vi "Set Controls Enable or Disable State Crop Utility.vi"(8 "error in (no error)":errorcluster, 10 "State":T1, 11 "Frame Grabber Data In":T2={"Camera Session"="", "Frame"=refnum, "AVI Refnum"=refnum, "Codecs"=[], "Frame number"=0, "Tracking File Refnum"=refnum, "Tick Count"=0, "Probe Object"=refnum, "Playback Probe Data"=[], "Rigid Body"={"Position"={"x (mm)"=0.0, "y (mm)"=0.0, "z (mm)"=0.0}, "Orientation"={"Pitch (rad)"=0.0, "Yaw (rad)"=0.0, "Roll (rad)"=0.0}, "Quaternion"={"qx"=0.0, "qy"=0.0, "qz"=0.0, "qw"=0.0}, "Tracked?"=FALSE}, "Total no frames playback"=0, "Video FPS"=0.0, "Camera connected?"=FALSE, "Scene"=refnum, "Cropped Frame"=refnum, "Tracker FPS"=0.0, "Crop ROI"=[], "Presentation Values"=[], "Elapsed time (ms)"=0, "Camera frames playback"=0, "Refnums"={"Live Refnum"=refnum, "Record Refnum"=refnum, "Playback Refnum"=refnum, "Frame Slider Refnum"=refnum, "Pause Refnum"=refnum, "Home Refnum"=refnum, "Set Crop Refnum"=refnum, "Clear Crop Refnum"=refnum, "stop refnum"=refnum, "Playback Rate Refnum"=refnum, "Presentation Refnum"=refnum, "Crop Time Frame Slider Refnum"=refnum, "Cancel Save Refnum"=refnum, "Reverse Playback Refnum"=refnum, "Recording Settings Refnum"=refnum, "Continuous Playback Refnum"=refnum, "Annotation Refnum"=refnum, "Export All Refnum"=refnum, "Export List Refnum"=refnum, "Fill List Refnum"=refnum, "Save Crop Refnum"=refnum, "Skip Forward Refnum"=refnum, "Skip Backward Refnum"=refnum, "Single Annotation Refnum"=refnum, "Load Video Refnum"=refnum, "Set Start Refnum"=refnum, "Set End Refnum"=refnum, "Add to List Refnum"=refnum, "List of Annotations Refnum"=refnum, "Camera Frame Refnum"=refnum, "Load Image Refnum"=refnum, "Saving Refnum"=refnum}, "Dimensions"={"Probe Dimensions"={"Probe Width"=0.0, "Probe Depth"=0.0, "Probe Height"=0.0}, "Room Dimensions"={"Room Width"=0.0, "Room Depth"=0.0, "Room Height"=0.0}}, "Playback Data As Strings"=[], "Cropped Tracking File Refnum"=refnum, "Cropped AVI Refnum"=refnum, "Header"=[], "Total euclidian distance"=0.0, "Annotation File Path"=path "", "Playback File Path"=path "", "Size per frame"=0.0, "Ground Truth File Refnum"=refnum, "Annotation Array"=[], "Annotation TIFFs Folder"=path "", "overwriting open file?"=FALSE, "Image Sequence"=[], "Video/Image Flag"=enum."Playback Video Frame", "Image sequence?"=FALSE, "Image sequence filenames"=[]}) -> (0 "error out":errorcluster)   [LabVIEW 2017]
uses:
  Controls/Frame Grabber Data.ctl
  <vilib>/userdefined/High Color/IMAQdx.ctl
  <vilib>/vision/Image Controls.llb/IMAQ Image.ctl
  <vilib>/vision/Avi.llb/IMAQ AVI2 Refnum.ctl
  Controls/Rigid Body Info.ctl
  Controls/Position.ctl
  Controls/Orientation.ctl
  Controls/Refnums.ctl
  Controls/Recording Settings.ctl
  Controls/Operator Settings.ctl
  Controls/Operator.ctl
  Controls/Patient Settings.ctl
  Controls/Dimensions.ctl
  Controls/Room Dimensions.ctl
  Controls/Crop Video State.ctl
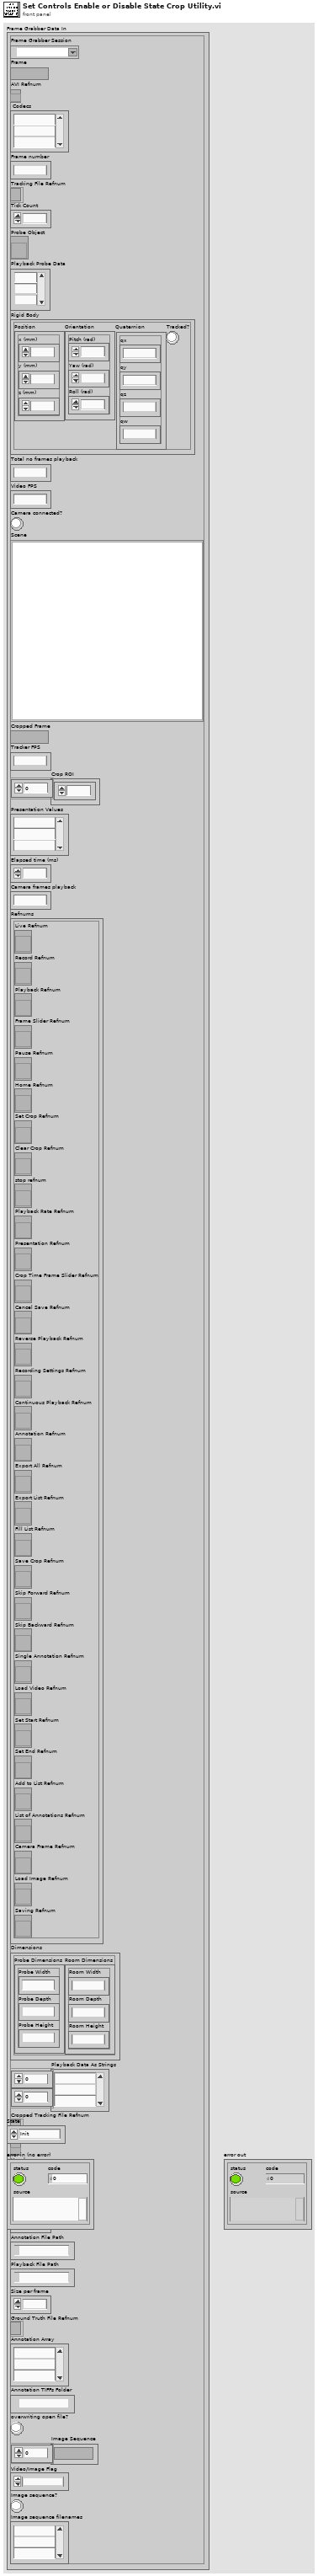
[diagram p1: front panel]
types:
  T1 = typedef "Crop Video State.ctl" = enum16{"Init", "Wait", "Load Image", "Load Video", "Play/Pause", "Playback Video Frame", "Display Image", "Save Image Sequence", "Save Video", "Export List", "Export All", "Close", "Set Crop Area", "Reset Crop Area", "Crop Inside", "Crop Outside", "Multi-Crop", "Re-Open Files", "Annotate Frame", "Annotate Clip", "Add to List", "Fill List", "Set Start", "Set End", "Error Handling", "Shutdown"}
  T2 = typedef "Frame Grabber Data.ctl" = cluster{"Camera Session":T3, "Frame":T4, "AVI Refnum":T5, "Codecs":string[], "Frame number":u32, "Tracking File Refnum":refnum<file>, "Tick Count":u32, "Probe Object":refnum<vi>, "Playback Probe Data":dbl[][], "Rigid Body":T6, "Total no frames playback":i32, "Video FPS":dbl, "Camera connected?":bool, "Scene":refnum<vi>, "Cropped Frame":T4, "Tracker FPS":dbl, "Crop ROI":i32[], "Presentation Values":string[], "Elapsed time (ms)":u32, "Camera frames playback":u32, "Refnums":T9, "Dimensions":T10, "Playback Data As Strings":string[][], "Cropped Tracking File Refnum":refnum<file>, "Cropped AVI Refnum":T5, "Header":string[], "Total euclidian distance":dbl, "Annotation File Path":path, "Playback File Path":path, "Size per frame":dbl, "Ground Truth File Refnum":refnum<file>, "Annotation Array":string[], "Annotation TIFFs Folder":path, "overwriting open file?":bool, "Image Sequence":T4[], "Video/Image Flag":T1, "Image sequence?":bool, "Image sequence filenames":string[]}
  T3 = typedef "IMAQdx.ctl" = refnum<k21>
  T4 = typedef "IMAQ Image.ctl" = refnum<image>
  T5 = typedef "IMAQ AVI2 Refnum.ctl" = refnum<k20>
  T6 = typedef "Rigid Body Info.ctl" = cluster{"Position":T7, "Orientation":T8, "Quaternion":cluster{"qx":sgl, "qy":sgl, "qz":sgl, "qw":sgl}, "Tracked?":bool}
  T7 = typedef "Position.ctl" = cluster{"x (mm)":sgl, "y (mm)":sgl, "z (mm)":sgl}
  T8 = typedef "Orientation.ctl" = cluster{"Pitch (rad)":sgl, "Yaw (rad)":sgl, "Roll (rad)":sgl}
  T9 = typedef "Refnums.ctl" = cluster{"Live Refnum":refnum<vi>, "Record Refnum":refnum<vi>, "Playback Refnum":refnum<vi>, "Frame Slider Refnum":refnum<vi>, "Pause Refnum":refnum<vi>, "Home Refnum":refnum<vi>, "Set Crop Refnum":refnum<vi>, "Clear Crop Refnum":refnum<vi>, "stop refnum":refnum<vi>, "Playback Rate Refnum":refnum<vi>, "Presentation Refnum":refnum<vi>, "Crop Time Frame Slider Refnum":refnum<vi>, "Cancel Save Refnum":refnum<vi>, "Reverse Playback Refnum":refnum<vi>, "Recording Settings Refnum":refnum<vi>, "Continuous Playback Refnum":refnum<vi>, "Annotation Refnum":refnum<vi>, "Export All Refnum":refnum<vi>, "Export List Refnum":refnum<vi>, "Fill List Refnum":refnum<vi>, "Save Crop Refnum":refnum<vi>, "Skip Forward Refnum":refnum<vi>, "Skip Backward Refnum":refnum<vi>, "Single Annotation Refnum":refnum<vi>, "Load Video Refnum":refnum<vi>, "Set Start Refnum":refnum<vi>, "Set End Refnum":refnum<vi>, "Add to List Refnum":refnum<vi>, "List of Annotations Refnum":refnum<vi>, "Camera Frame Refnum":refnum<vi>, "Load Image Refnum":refnum<vi>, "Saving Refnum":refnum<vi>}
  T10 = typedef "Dimensions.ctl" = cluster{"Probe Dimensions":cluster{"Probe Width":sgl, "Probe Depth":sgl, "Probe Height":sgl}, "Room Dimensions":T11}
  T11 = typedef "Room Dimensions.ctl" = cluster{"Room Width":dbl, "Room Depth":dbl, "Room Height":dbl}
  T12 = enum8{"Enabled", "Disabled", "Disabled and Grayed Out"}
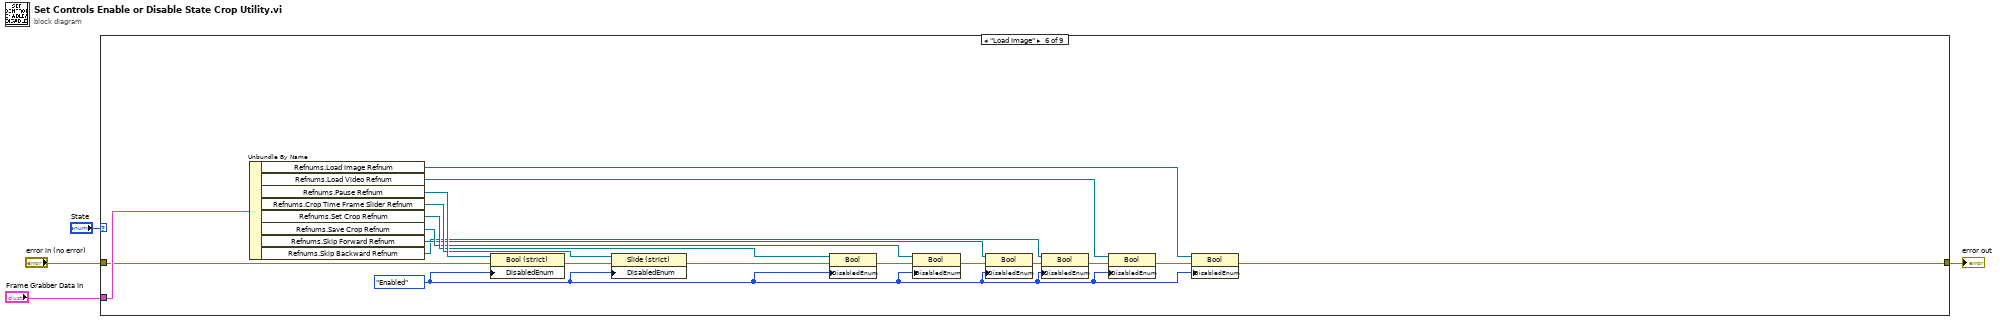
[diagram p0: block diagram]
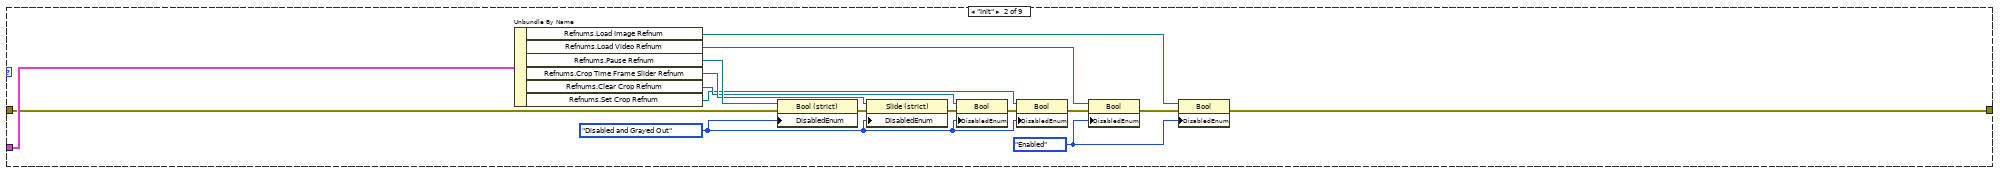
[diagram p3: hidden frame]
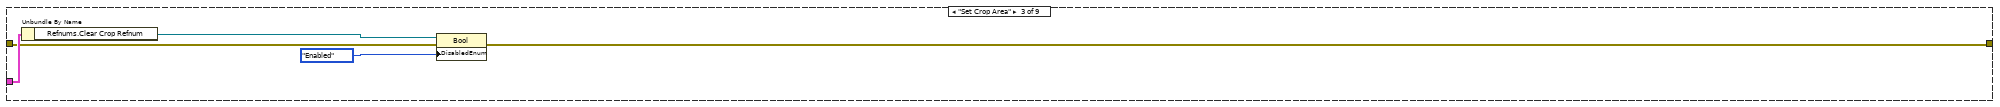
[diagram p4: hidden frame]
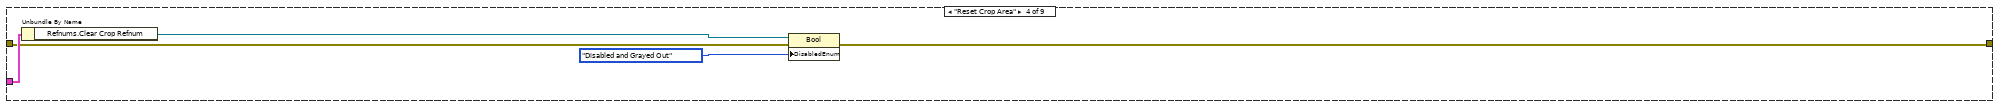
[diagram p5: hidden frame]
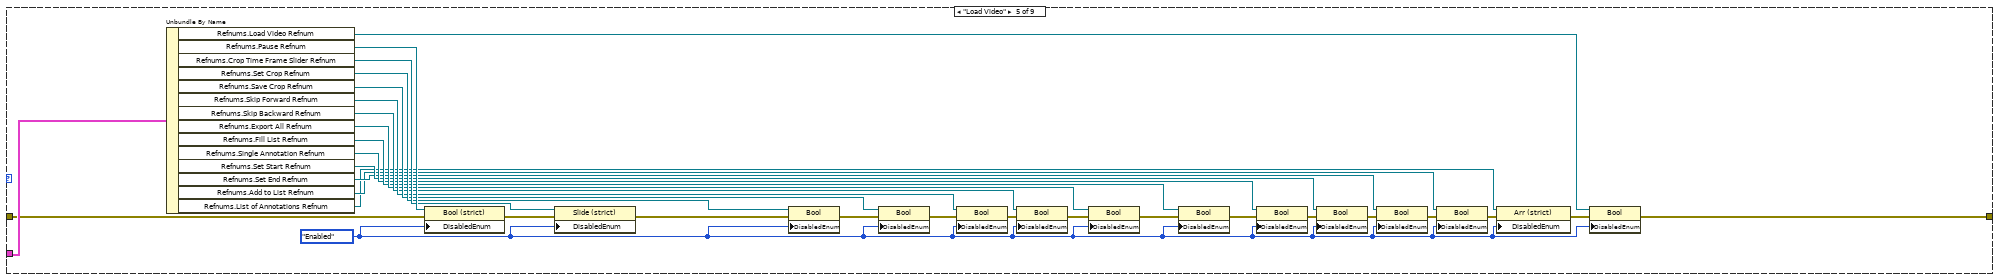
[diagram p6: hidden frame]
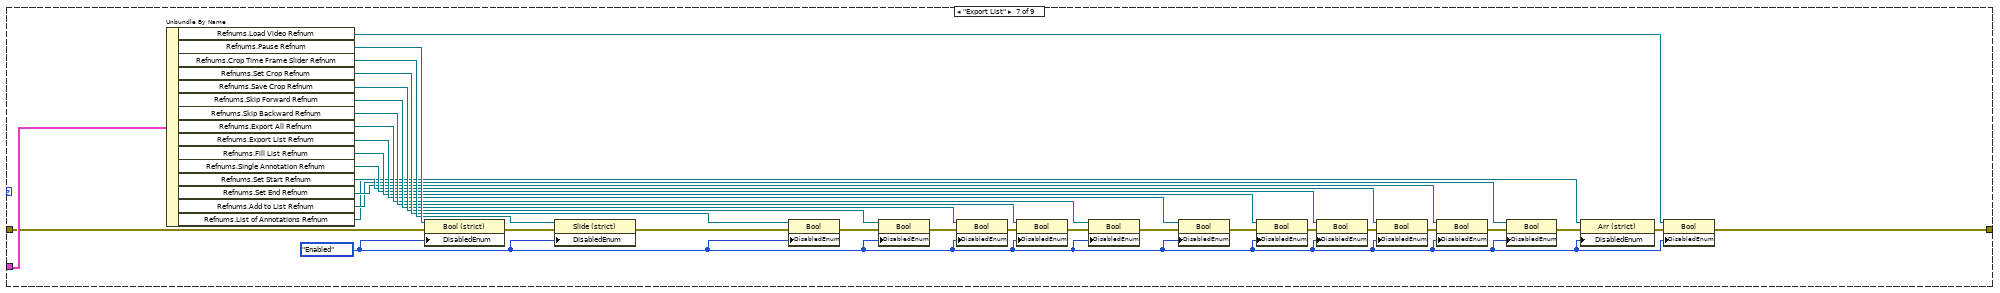
[diagram p7: hidden frame]
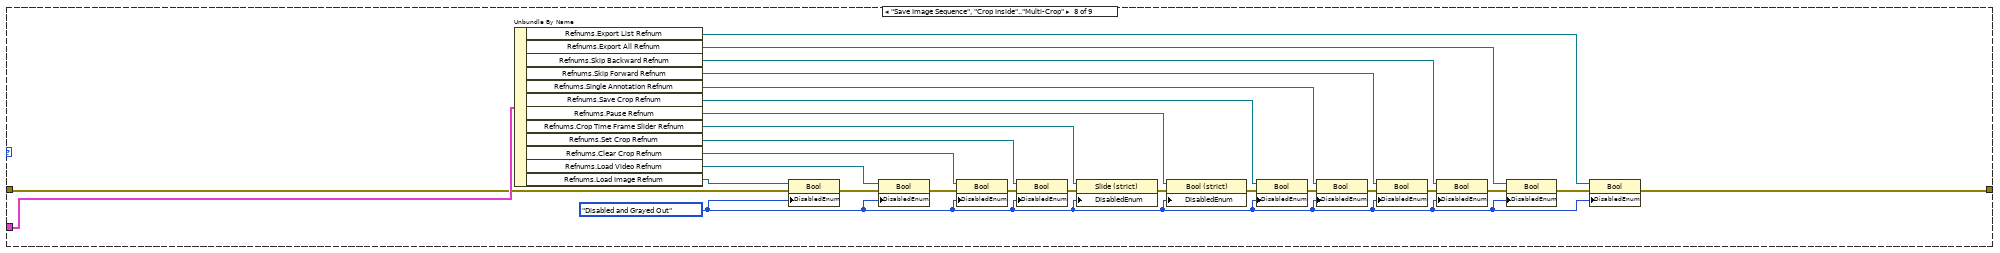
[diagram p8: hidden frame]
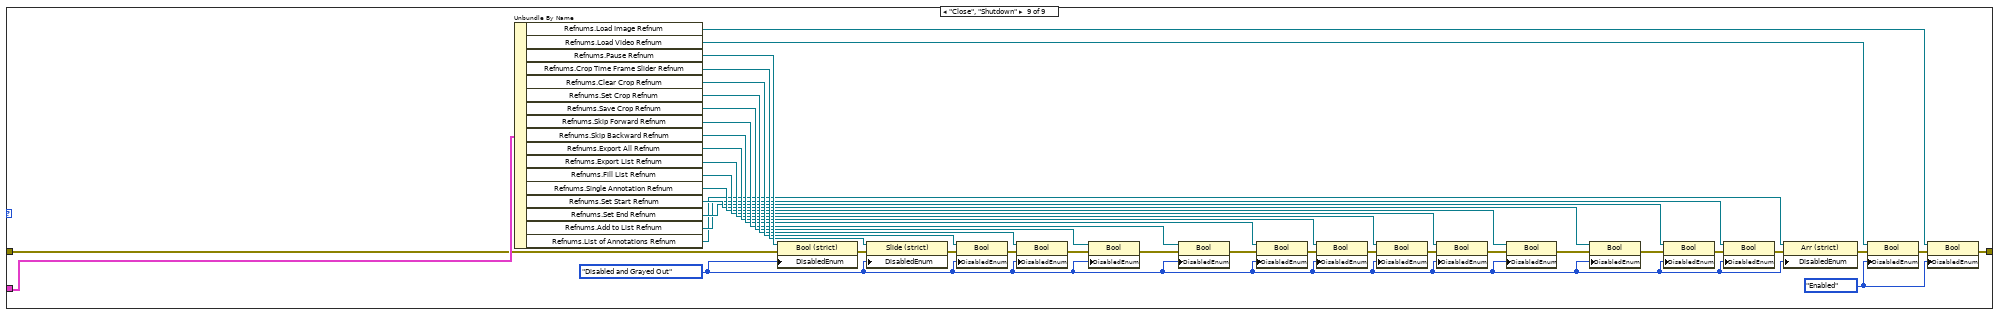
[diagram p9: hidden frame]
diagram:
  n1 = case shown="\"Load Image\"" "State" {
    tunnel: "Frame Grabber Data In" -> [_ w21 w26 w31 w62 w81 w114 w141 w179]
    tunnel: "error in (no error)" -> [w5 w17 w23 w28 w58 w77 w110 w116 w175]
    tunnel: [w5 w6 w22 w27 w32 w64 w82 w119 w143] -> w2
    frame Default {
    }
    frame "Init" {
      w8 = T12."Enabled" ("Disabled")
      w14 = T12."Disabled and Grayed Out" ("Disabled")
      n2 = Unbundle By Name(w21) -> ("Refnums.Load Image Refnum"=w7:refnum<vi>, "Refnums.Load Video Refnum"=w11:refnum<vi>, "Refnums.Pause Refnum"=w20:refnum<vi>, "Refnums.Crop Time Frame Slider Refnum"=w19:refnum<vi>, "Refnums.Clear Crop Refnum"=w16:refnum<vi>, "Refnums.Set Crop Refnum"=w15:refnum<vi>)
      n3 = property class="Bool (strict)"(reference=w20, error in=w17, "DisabledEnum"=w14) -> (error out=w18:errorcluster)  [unwired: 1 out]
      n4 = property class="Slide (strict)"(reference=w19, error in=w18, "DisabledEnum"=w14) -> (error out=w13:errorcluster)  [unwired: 1 out]
      n5 = property class="Bool"(reference=w16, error in=w13, "DisabledEnum"=w14) -> (error out=w12:errorcluster)  [unwired: 1 out]
      n6 = property class="Bool"(reference=w15, error in=w12, "DisabledEnum"=w14) -> (error out=w10:errorcluster)  [unwired: 1 out]
      n7 = property class="Bool"(reference=w11, error in=w10, "DisabledEnum"=w8) -> (error out=w9:errorcluster)  [unwired: 1 out]
      n8 = property class="Bool"(reference=w7, error in=w9, "DisabledEnum"=w8) -> (error out=w6:errorcluster)  [unwired: 1 out]
    }
    frame "Set Crop Area" {
      n9 = Unbundle By Name(w26) -> ("Refnums.Clear Crop Refnum"=w25:refnum<vi>)
      n10 = property class="Bool"(reference=w25, error in=w23, "DisabledEnum"=T12."Enabled" ("Disabled")) -> (error out=w22:errorcluster)  [unwired: 1 out]
    }
    frame "Reset Crop Area" {
      n11 = Unbundle By Name(w31) -> ("Refnums.Clear Crop Refnum"=w30:refnum<vi>)
      n12 = property class="Bool"(reference=w30, error in=w28, "DisabledEnum"=T12."Disabled and Grayed Out" ("Disabled")) -> (error out=w27:errorcluster)  [unwired: 1 out]
    }
    frame "Load Video" {
      w34 = T12."Enabled" ("Disabled")
      n13 = Unbundle By Name(w62) -> ("Refnums.Load Video Refnum"=w35:refnum<vi>, "Refnums.Pause Refnum"=w61:refnum<vi>, "Refnums.Crop Time Frame Slider Refnum"=w60:refnum<vi>, "Refnums.Set Crop Refnum"=w57:refnum<vi>, "Refnums.Save Crop Refnum"=w54:refnum<vi>, "Refnums.Skip Forward Refnum"=w53:refnum<vi>, "Refnums.Skip Backward Refnum"=w52:refnum<vi>, "Refnums.Export All Refnum"=w49:refnum<vi>, "Refnums.Fill List Refnum"=w46:refnum<vi>, "Refnums.Single Annotation Refnum"=w45:refnum<vi>, "Refnums.Set Start Refnum"=w39:refnum<vi>, "Refnums.Set End Refnum"=w38:refnum<vi>, "Refnums.Add to List Refnum"=w37:refnum<vi>, "Refnums.List of Annotations Refnum"=w36:refnum<vi>)
      n14 = property class="Bool (strict)"(reference=w61, error in=w58, "DisabledEnum"=w34) -> (error out=w59:errorcluster)  [unwired: 1 out]
      n15 = property class="Slide (strict)"(reference=w60, error in=w59, "DisabledEnum"=w34) -> (error out=w56:errorcluster)  [unwired: 1 out]
      n16 = property class="Bool"(reference=w57, error in=w56, "DisabledEnum"=w34) -> (error out=w55:errorcluster)  [unwired: 1 out]
      n17 = property class="Bool"(reference=w54, error in=w55, "DisabledEnum"=w34) -> (error out=w51:errorcluster)  [unwired: 1 out]
      n18 = property class="Bool"(reference=w53, error in=w51, "DisabledEnum"=w34) -> (error out=w50:errorcluster)  [unwired: 1 out]
      n19 = property class="Bool"(reference=w52, error in=w50, "DisabledEnum"=w34) -> (error out=w48:errorcluster)  [unwired: 1 out]
      n20 = property class="Bool"(reference=w49, error in=w48, "DisabledEnum"=w34) -> (error out=w47:errorcluster)  [unwired: 1 out]
      n21 = property class="Bool"(reference=w46, error in=w47, "DisabledEnum"=w34) -> (error out=w44:errorcluster)  [unwired: 1 out]
      n22 = property class="Bool"(reference=w45, error in=w44, "DisabledEnum"=w34) -> (error out=w41:errorcluster)  [unwired: 1 out]
      n23 = property class="Bool"(reference=w39, error in=w41, "DisabledEnum"=w34) -> (error out=w42:errorcluster)  [unwired: 1 out]
      n24 = property class="Bool"(reference=w38, error in=w42, "DisabledEnum"=w34) -> (error out=w43:errorcluster)  [unwired: 1 out]
      n25 = property class="Bool"(reference=w37, error in=w43, "DisabledEnum"=w34) -> (error out=w40:errorcluster)  [unwired: 1 out]
      n26 = property class="Arr (strict)"(reference=w36, error in=w40, "DisabledEnum"=w34) -> (error out=w33:errorcluster)  [unwired: 1 out]
      n27 = property class="Bool"(reference=w35, error in=w33, "DisabledEnum"=w34) -> (error out=w32:errorcluster)  [unwired: 1 out]
    }
    frame "Load Image" {
      w65 = T12."Enabled" ("Disabled")
      n28 = Unbundle By Name(w81) -> ("Refnums.Load Image Refnum"=w63:refnum<vi>, "Refnums.Load Video Refnum"=w67:refnum<vi>, "Refnums.Pause Refnum"=w80:refnum<vi>, "Refnums.Crop Time Frame Slider Refnum"=w79:refnum<vi>, "Refnums.Set Crop Refnum"=w76:refnum<vi>, "Refnums.Save Crop Refnum"=w73:refnum<vi>, "Refnums.Skip Forward Refnum"=w72:refnum<vi>, "Refnums.Skip Backward Refnum"=w71:refnum<vi>)
      n29 = property class="Bool (strict)"(reference=w80, error in=w77, "DisabledEnum"=w65) -> (error out=w78:errorcluster)  [unwired: 1 out]
      n30 = property class="Slide (strict)"(reference=w79, error in=w78, "DisabledEnum"=w65) -> (error out=w75:errorcluster)  [unwired: 1 out]
      n31 = property class="Bool"(reference=w76, error in=w75, "DisabledEnum"=w65) -> (error out=w74:errorcluster)  [unwired: 1 out]
      n32 = property class="Bool"(reference=w73, error in=w74, "DisabledEnum"=w65) -> (error out=w70:errorcluster)  [unwired: 1 out]
      n33 = property class="Bool"(reference=w72, error in=w70, "DisabledEnum"=w65) -> (error out=w69:errorcluster)  [unwired: 1 out]
      n34 = property class="Bool"(reference=w71, error in=w69, "DisabledEnum"=w65) -> (error out=w68:errorcluster)  [unwired: 1 out]
      n35 = property class="Bool"(reference=w67, error in=w68, "DisabledEnum"=w65) -> (error out=w66:errorcluster)  [unwired: 1 out]
      n36 = property class="Bool"(reference=w63, error in=w66, "DisabledEnum"=w65) -> (error out=w64:errorcluster)  [unwired: 1 out]
    }
    frame "Export List" {
      w84 = T12."Enabled" ("Disabled")
      n37 = Unbundle By Name(w114) -> ("Refnums.Load Video Refnum"=w85:refnum<vi>, "Refnums.Pause Refnum"=w113:refnum<vi>, "Refnums.Crop Time Frame Slider Refnum"=w112:refnum<vi>, "Refnums.Set Crop Refnum"=w109:refnum<vi>, "Refnums.Save Crop Refnum"=w106:refnum<vi>, "Refnums.Skip Forward Refnum"=w105:refnum<vi>, "Refnums.Skip Backward Refnum"=w104:refnum<vi>, "Refnums.Export All Refnum"=w101:refnum<vi>, "Refnums.Export List Refnum"=w100:refnum<vi>, "Refnums.Fill List Refnum"=w96:refnum<vi>, "Refnums.Single Annotation Refnum"=w95:refnum<vi>, "Refnums.Set Start Refnum"=w89:refnum<vi>, "Refnums.Set End Refnum"=w88:refnum<vi>, "Refnums.Add to List Refnum"=w87:refnum<vi>, "Refnums.List of Annotations Refnum"=w86:refnum<vi>)
      n38 = property class="Bool (strict)"(reference=w113, error in=w110, "DisabledEnum"=w84) -> (error out=w111:errorcluster)  [unwired: 1 out]
      n39 = property class="Slide (strict)"(reference=w112, error in=w111, "DisabledEnum"=w84) -> (error out=w108:errorcluster)  [unwired: 1 out]
      n40 = property class="Bool"(reference=w109, error in=w108, "DisabledEnum"=w84) -> (error out=w107:errorcluster)  [unwired: 1 out]
      n41 = property class="Bool"(reference=w106, error in=w107, "DisabledEnum"=w84) -> (error out=w103:errorcluster)  [unwired: 1 out]
      n42 = property class="Bool"(reference=w105, error in=w103, "DisabledEnum"=w84) -> (error out=w102:errorcluster)  [unwired: 1 out]
      n43 = property class="Bool"(reference=w104, error in=w102, "DisabledEnum"=w84) -> (error out=w99:errorcluster)  [unwired: 1 out]
      n44 = property class="Bool"(reference=w101, error in=w99, "DisabledEnum"=w84) -> (error out=w98:errorcluster)  [unwired: 1 out]
      n45 = property class="Bool"(reference=w100, error in=w98, "DisabledEnum"=w84) -> (error out=w97:errorcluster)  [unwired: 1 out]
      n46 = property class="Bool"(reference=w96, error in=w97, "DisabledEnum"=w84) -> (error out=w94:errorcluster)  [unwired: 1 out]
      n47 = property class="Bool"(reference=w95, error in=w94, "DisabledEnum"=w84) -> (error out=w91:errorcluster)  [unwired: 1 out]
      n48 = property class="Bool"(reference=w89, error in=w91, "DisabledEnum"=w84) -> (error out=w92:errorcluster)  [unwired: 1 out]
      n49 = property class="Bool"(reference=w88, error in=w92, "DisabledEnum"=w84) -> (error out=w93:errorcluster)  [unwired: 1 out]
      n50 = property class="Bool"(reference=w87, error in=w93, "DisabledEnum"=w84) -> (error out=w90:errorcluster)  [unwired: 1 out]
      n51 = property class="Arr (strict)"(reference=w86, error in=w90, "DisabledEnum"=w84) -> (error out=w83:errorcluster)  [unwired: 1 out]
      n52 = property class="Bool"(reference=w85, error in=w83, "DisabledEnum"=w84) -> (error out=w82:errorcluster)  [unwired: 1 out]
    }
    frame "Save Image Sequence", "Crop Inside".."Multi-Crop" {
      w117 = T12."Disabled and Grayed Out" ("Disabled")
      n53 = Unbundle By Name(w141) -> ("Refnums.Export List Refnum"=w124:refnum<vi>, "Refnums.Export All Refnum"=w125:refnum<vi>, "Refnums.Skip Backward Refnum"=w126:refnum<vi>, "Refnums.Skip Forward Refnum"=w127:refnum<vi>, "Refnums.Single Annotation Refnum"=w130:refnum<vi>, "Refnums.Save Crop Refnum"=w131:refnum<vi>, "Refnums.Pause Refnum"=w136:refnum<vi>, "Refnums.Crop Time Frame Slider Refnum"=w137:refnum<vi>, "Refnums.Set Crop Refnum"=w138:refnum<vi>, "Refnums.Clear Crop Refnum"=w139:refnum<vi>, "Refnums.Load Video Refnum"=w140:refnum<vi>, "Refnums.Load Image Refnum"=w118:refnum<vi>)
      n54 = property class="Bool"(reference=w118, error in=w116, "DisabledEnum"=w117) -> (error out=w115:errorcluster)  [unwired: 1 out]
      n55 = property class="Bool"(reference=w140, error in=w115, "DisabledEnum"=w117) -> (error out=w135:errorcluster)  [unwired: 1 out]
      n56 = property class="Bool"(reference=w139, error in=w135, "DisabledEnum"=w117) -> (error out=w134:errorcluster)  [unwired: 1 out]
      n57 = property class="Bool"(reference=w138, error in=w134, "DisabledEnum"=w117) -> (error out=w133:errorcluster)  [unwired: 1 out]
      n58 = property class="Slide (strict)"(reference=w137, error in=w133, "DisabledEnum"=w117) -> (error out=w132:errorcluster)  [unwired: 1 out]
      n59 = property class="Bool (strict)"(reference=w136, error in=w132, "DisabledEnum"=w117) -> (error out=w129:errorcluster)  [unwired: 1 out]
      n60 = property class="Bool"(reference=w131, error in=w129, "DisabledEnum"=w117) -> (error out=w128:errorcluster)  [unwired: 1 out]
      n61 = property class="Bool"(reference=w130, error in=w128, "DisabledEnum"=w117) -> (error out=w123:errorcluster)  [unwired: 1 out]
      n62 = property class="Bool"(reference=w127, error in=w123, "DisabledEnum"=w117) -> (error out=w122:errorcluster)  [unwired: 1 out]
      n63 = property class="Bool"(reference=w126, error in=w122, "DisabledEnum"=w117) -> (error out=w121:errorcluster)  [unwired: 1 out]
      n64 = property class="Bool"(reference=w125, error in=w121, "DisabledEnum"=w117) -> (error out=w120:errorcluster)  [unwired: 1 out]
      n65 = property class="Bool"(reference=w124, error in=w120, "DisabledEnum"=w117) -> (error out=w119:errorcluster)  [unwired: 1 out]
    }
    frame "Close", "Shutdown" {
      w145 = T12."Enabled" ("Disabled")
      w152 = T12."Disabled and Grayed Out" ("Disabled")
      n66 = Unbundle By Name(w179) -> ("Refnums.Load Image Refnum"=w142:refnum<vi>, "Refnums.Load Video Refnum"=w160:refnum<vi>, "Refnums.Pause Refnum"=w178:refnum<vi>, "Refnums.Crop Time Frame Slider Refnum"=w177:refnum<vi>, "Refnums.Clear Crop Refnum"=w174:refnum<vi>, "Refnums.Set Crop Refnum"=w173:refnum<vi>, "Refnums.Save Crop Refnum"=w169:refnum<vi>, "Refnums.Skip Forward Refnum"=w168:refnum<vi>, "Refnums.Skip Backward Refnum"=w167:refnum<vi>, "Refnums.Export All Refnum"=w164:refnum<vi>, "Refnums.Export List Refnum"=w163:refnum<vi>, "Refnums.Fill List Refnum"=w159:refnum<vi>, "Refnums.Single Annotation Refnum"=w156:refnum<vi>, "Refnums.Set Start Refnum"=w150:refnum<vi>, "Refnums.Set End Refnum"=w149:refnum<vi>, "Refnums.Add to List Refnum"=w148:refnum<vi>, "Refnums.List of Annotations Refnum"=w147:refnum<vi>)
      n67 = property class="Bool (strict)"(reference=w178, error in=w175, "DisabledEnum"=w152) -> (error out=w176:errorcluster)  [unwired: 1 out]
      n68 = property class="Slide (strict)"(reference=w177, error in=w176, "DisabledEnum"=w152) -> (error out=w172:errorcluster)  [unwired: 1 out]
      n69 = property class="Bool"(reference=w174, error in=w172, "DisabledEnum"=w152) -> (error out=w171:errorcluster)  [unwired: 1 out]
      n70 = property class="Bool"(reference=w173, error in=w171, "DisabledEnum"=w152) -> (error out=w170:errorcluster)  [unwired: 1 out]
      n71 = property class="Bool"(reference=w169, error in=w170, "DisabledEnum"=w152) -> (error out=w166:errorcluster)  [unwired: 1 out]
      n72 = property class="Bool"(reference=w168, error in=w166, "DisabledEnum"=w152) -> (error out=w165:errorcluster)  [unwired: 1 out]
      n73 = property class="Bool"(reference=w167, error in=w165, "DisabledEnum"=w152) -> (error out=w162:errorcluster)  [unwired: 1 out]
      n74 = property class="Bool"(reference=w164, error in=w162, "DisabledEnum"=w152) -> (error out=w161:errorcluster)  [unwired: 1 out]
      n75 = property class="Bool"(reference=w163, error in=w161, "DisabledEnum"=w152) -> (error out=w158:errorcluster)  [unwired: 1 out]
      n76 = property class="Bool"(reference=w159, error in=w158, "DisabledEnum"=w152) -> (error out=w157:errorcluster)  [unwired: 1 out]
      n77 = property class="Bool"(reference=w156, error in=w157, "DisabledEnum"=w152) -> (error out=w146:errorcluster)  [unwired: 1 out]
      n78 = property class="Bool"(reference=w150, error in=w146, "DisabledEnum"=w152) -> (error out=w154:errorcluster)  [unwired: 1 out]
      n79 = property class="Bool"(reference=w149, error in=w154, "DisabledEnum"=w152) -> (error out=w155:errorcluster)  [unwired: 1 out]
      n80 = property class="Bool"(reference=w148, error in=w155, "DisabledEnum"=w152) -> (error out=w153:errorcluster)  [unwired: 1 out]
      n81 = property class="Arr (strict)"(reference=w147, error in=w153, "DisabledEnum"=w152) -> (error out=w151:errorcluster)  [unwired: 1 out]
      n82 = property class="Bool"(reference=w160, error in=w151, "DisabledEnum"=w145) -> (error out=w144:errorcluster)  [unwired: 1 out]
      n83 = property class="Bool"(reference=w142, error in=w144, "DisabledEnum"=w145) -> (error out=w143:errorcluster)  [unwired: 1 out]
    }
  }
  "error out" <- w2
